vi "Init Main UI.vi"(8 "error in (no error)":errorcluster, 11 "GVIWebProcessorApp in":refnum<class "GVIWebProcessorApp.lvclass">) -> (0 "error out":errorcluster, 3 "GVIWebProcessorApp out":refnum<class "GVIWebProcessorApp.lvclass">)   [LabVIEW 2020, in "PicoG-Processor.lvlib" / "GVIWebProcessorApp.lvclass"]
uses:
  GVIWebProcessorApp.lvclass
  Builds/picoG/ppl/PicoG-Core.lvlibp/PicoG-Processor/PicoG-Core/PlatformPluginManager/PlatformPluginManager.lvclass
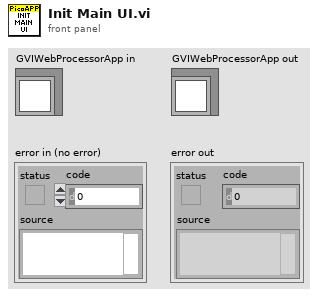
[diagram p1: front panel]
types:
  T1 = typedef "PicoG-Processor.lvlib/GVIWebProcessorApp.lvclass/UI Refs.ctl" = cluster{"Main Window":refnum<vi>, "List Panel":refnum<vi>, "H Splitter":refnum<vi>, "V Splitter":refnum<vi>, "Open Project":refnum<vi>, "Project Name":refnum<vi>, "Auto Process":refnum<vi>, "Auto Deploy":refnum<vi>, "Process Platform":refnum<vi>, "Last Target":refnum<vi>}
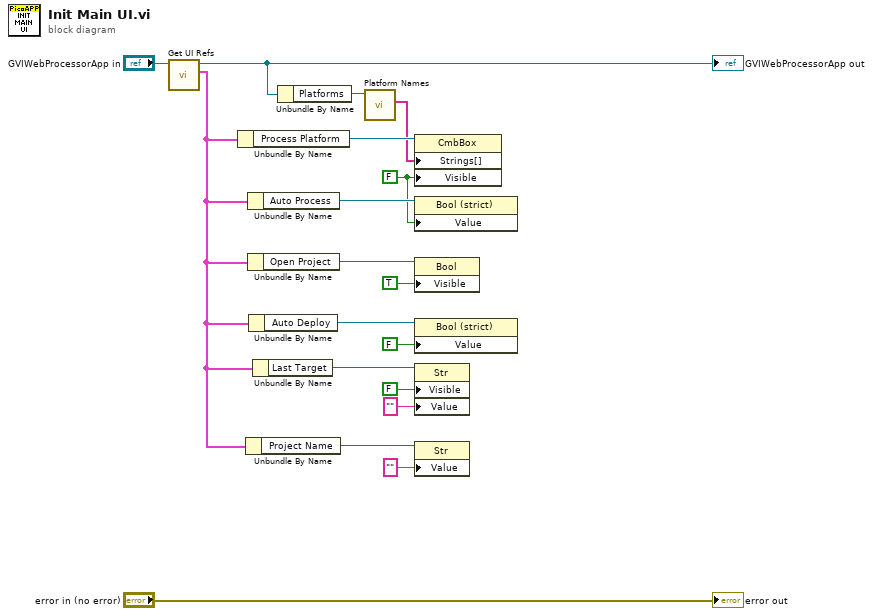
[diagram p0: block diagram]
diagram:
  w11 = FALSE ("Visible")
  n1 = call "Get UI Refs.vi"("GVIWebProcessorApp in"="GVIWebProcessorApp in") -> ("UI Refs"=w3:T1, "GVIWebProcessorApp out"=w16:refnum<class "GVIWebProcessorApp.lvclass">)  [unwired: 8 in, 1 out]
  "GVIWebProcessorApp out" <- w16
  n2 = Unbundle By Name(w3) -> ("Process Platform"=w14:refnum<vi>)
  n3 = Unbundle By Name(w3) -> ("Project Name"=w4:refnum<vi>)
  n4 = Unbundle By Name(w3) -> ("Auto Process"=w12:refnum<vi>)
  n5 = Unbundle By Name(w3) -> ("Open Project"=w10:refnum<vi>)
  n6 = Unbundle By Name(w3) -> ("Auto Deploy"=w6:refnum<vi>)
  n7 = Unbundle By Name(w3) -> ("Last Target"=w5:refnum<vi>)
  n8 = Unbundle By Name(w16) -> ("Platforms"=w15:refnum<class "PlatformPluginManager.lvclass">)
  n9 = call "Platform Names.vi"("TargetPluginManager in"=w15) -> ("Platforms"=w13:string[])  [unwired: 8 in, 2 out]
  n10 = property class="CmbBox"(reference=w14, "Strings[]"=w13, "Visible"=w11) -> ()  [unwired: 1 in, 2 out]
  n11 = property class="Bool (strict)"(reference=w12, "Value"=w11) -> ()  [unwired: 1 in, 2 out]
  n12 = property class="Bool"(reference=w10, "Visible"=TRUE) -> ()  [unwired: 1 in, 2 out]
  n13 = property class="Bool (strict)"(reference=w6, "Value"=FALSE) -> ()  [unwired: 1 in, 2 out]
  n14 = property class="Str"(reference=w5, "Visible"=FALSE, "Value"="") -> ()  [unwired: 1 in, 2 out]
  n15 = property class="Str"(reference=w4, "Value"="") -> ()  [unwired: 1 in, 2 out]
  "error out" <- "error in (no error)"
